vi "CheckBatteryColor.vi"(10 "input cluster":T2, 11 "Image In":T1) -> (2 "OK":bool, 3 "Image Out":T1)   [LabVIEW 2019]
uses:
  <vilib>/vision/Image Controls.llb/IMAQ Image.ctl
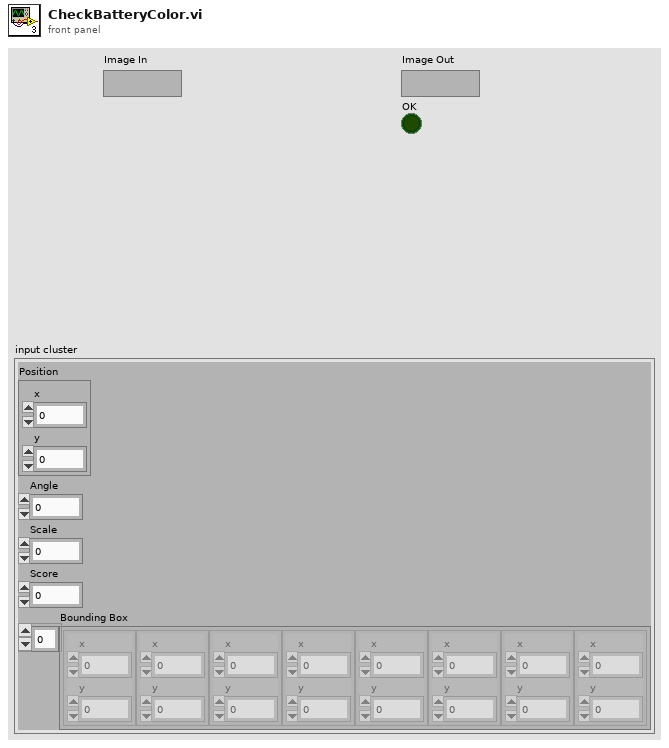
[diagram p1: front panel]
types:
  T1 = typedef "IMAQ Image.ctl" = refnum<image>
  T2 = cluster{"Position":cluster{"x":sgl, "y":sgl}, "Angle":sgl, "Scale":sgl, "Score":sgl, "Bounding Box":cluster{"x":sgl, "y":sgl}[]}
  T3 = typedef "IMAQ Rectangle" = cluster{"Left":i32, "Top":i32, "Right":i32, "Bottom":i32, "Rotation":dbl}
  T4 = typedef "ROI Descriptor" = cluster{"Global Rectangle":i32[], "Contours":cluster{"ID":enum32{"External", "Internal"}, "Type":u32, "Coordinates":i32[]}[]}
  T5 = cluster{"Minimal Value":sgl, "Maximal Value":sgl, "Mean Value":sgl, "Standard  Variation":sgl, "Area (pixels)":i32}
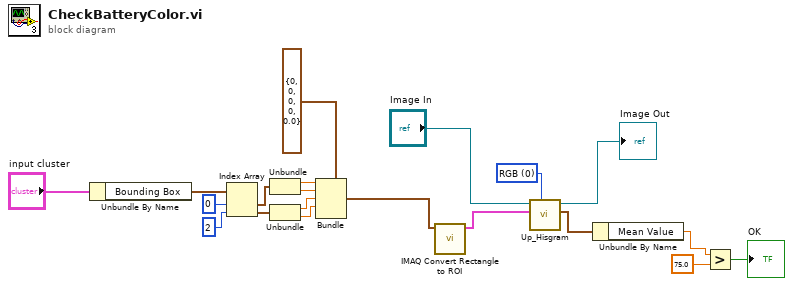
[diagram p0: block diagram]
diagram:
  w17 = u16 0 items=["RGB", "HSL", "HSV", "HSI"] ("Color Mode")
  n1 = Unbundle By Name("input cluster") -> ("Bounding Box"=w20:cluster{"x":sgl, "y":sgl}[])
  n2 = Index Array(array=w20, index #1=0 ("index"), index #2=2 ("index")) -> (element #1=w15:cluster{"x":sgl, "y":sgl}, element #2=w14:cluster{"x":sgl, "y":sgl})
  n3 = Unbundle(w15) -> ("x"=w13:sgl, "y"=w12:sgl)
  n4 = Unbundle(w14) -> ("x"=w11:sgl, "y"=w10:sgl)
  n5 = Bundle(cluster=T3 {"Left"=0, "Top"=0, "Right"=0, "Bottom"=0, "Rotation"=0.0} ("Rectangle"), "Left"=w13, "Top"=w12, "Right"=w11, "Bottom"=w10) -> (w8:T3)  [unwired: 1 in]
  n6 = call "IMAQ Convert Rectangle to ROI"("Rectangle"=w8) -> ("ROI Descriptor"=w7:T4)  [unwired: 8 in, 1 out]
  n7 = call "Up_Hisgram.vi"("Color Mode"=w17, "ROI Descriptor"=w7, "Image In"="Image In") -> ("Statistics"=w4:T5, "Image Out"=→"Image Out":T1)  [unwired: 5 in, 2 out]
  n8 = Unbundle By Name(w4) -> ("Mean Value"=w3:sgl)
  n9 = Greater?(x=w3, y=sgl 75.0) -> (0:→"OK":bool)
